vi "Create folder path if needed and file from file path.vi"(8 "error in":errorcluster, 11 "String file path":string) -> (0 "error out":errorcluster, 2 "file path":path, 3 "New file refnum":refnum<file>)   [LabVIEW 2013]
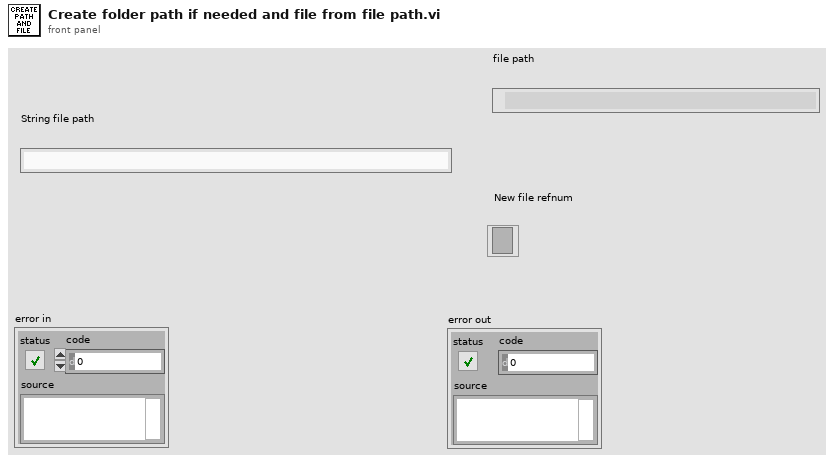
[diagram p1: front panel]
types:
  T1 = enum16{"open", "replace", "create", "open or create", "replace or create", "replace or create with confirmation"}
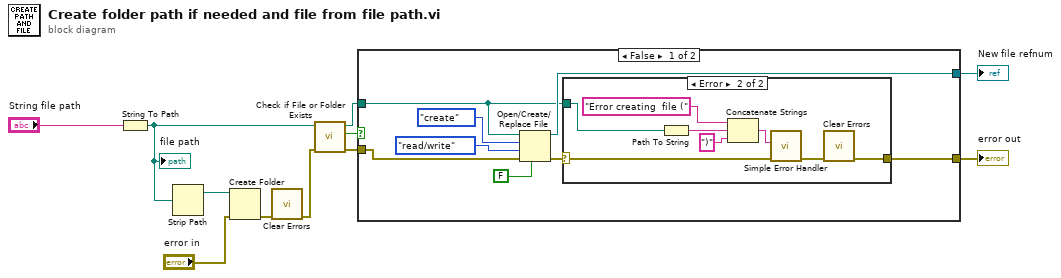
[diagram p0: block diagram]
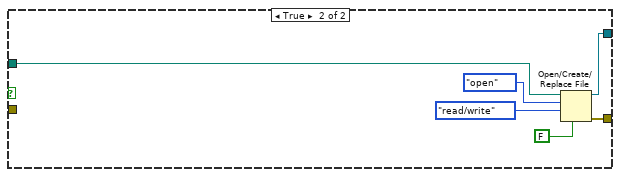
[diagram p3: hidden frame]
diagram:
  n1 = String To Path(string="String file path") -> (path=w8:path)
  "file path" <- w8
  n2 = Strip Path(path=w8) -> (stripped path=w10:path)  [unwired: 1 out]
  n3 = Create Folder(path (use dialog)=w10, error in="error in") -> (error out=w6:errorcluster)  [unwired: 1 in, 2 out]
  n4 = call <vilib>:"Clear Errors.vi"("error in (no error)"=w6) -> ("error out"=w5:errorcluster)  [unwired: 6 in]
  n5 = call <vilib>:"Check if File or Folder Exists.vi"("error in (no error)"=w5, "path"=w8) -> ("error out"=w2:errorcluster, "file or folder exists?"=w3:bool, "dup path"=w4:path)  [unwired: 7 in]
  n6 = case shown="False" w3 {
    tunnel: w4 -> [w13 w34]
    tunnel: [w14 w32] -> w11
    tunnel: [w17 w33] -> w1
    tunnel: w2 -> [w12 _]
    frame False {
      n7 = Open/Create/Replace File(file path (use dialog)=w13, error in=w12, operation (0:open)=T1."create", access (0:read/write)=enum16{"read/write", "read-only", "write-only"}."read/write", disable buffering (F)=FALSE) -> (refnum out=w17:refnum<file>, error out=w15:errorcluster)  [unwired: 1 in, 1 out]
      n8 = case shown="Error" w15 {
        selector: w15 -> [w20 w23]
        tunnel: [w20 w28] -> w14
        tunnel: w13 -> [_ w25]
        frame No Error {
        }
        frame Error {
          n9 = Path To String(path=w25) -> (string=w24:string)
          n10 = Concatenate Strings("Error creating  file (" ("message"), w24, ")" ("string")) -> (w21:string)
          n11 = call <vilib>:"Simple Error Handler.vi"("error source (\" \")"=w21, "error in (no error)"=w23) -> ("error out"=w22:errorcluster)  [unwired: 3 in, 4 out]
          n12 = call <vilib>:"Clear Errors.vi"("error in (no error)"=w22) -> ("error out"=w28:errorcluster)  [unwired: 6 in]
        }
      }
    }
    frame True {
      n13 = Open/Create/Replace File(file path (use dialog)=w34, operation (0:open)=T1."open", access (0:read/write)=enum16{"read/write", "read-only", "write-only"}."read/write", disable buffering (F)=FALSE) -> (refnum out=w33:refnum<file>, error out=w32:errorcluster)  [unwired: 2 in, 1 out]
    }
  }
  "error out" <- w11
  "New file refnum" <- w1
